vi "AllPath.vi"() -> ()   [LabVIEW 2018]
panel:
  out "路径":T1
  # "路径"
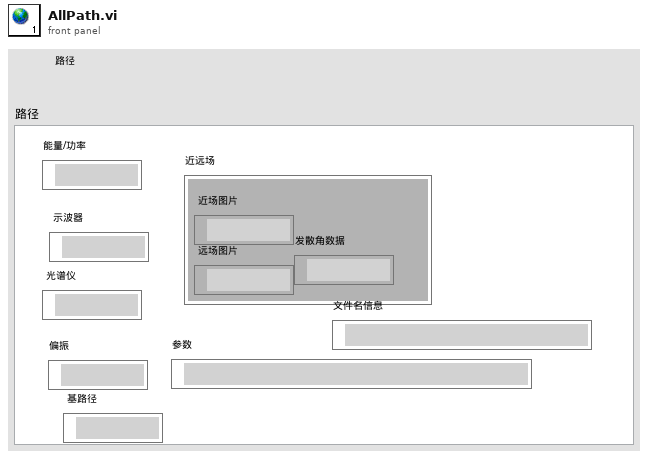
[diagram p1: front panel]
types:
  T1 = cluster{"能量/功率":path, " 示波器":path, " 光谱仪":path, "偏振":path, "近远场":cluster{" 近场图片":path, " 远场图片":path, "发散角数据":path}, "参数":path, " 基路径":path, "文件名信息":path}
diagram:
